vi "Write logEntry.vi"(10 "logEntry":string[](array[string]), 11 "Logger in":refnum<class "Log.lvclass">) -> (3 "Logger out":refnum<class "Log.lvclass">)   [LabVIEW 2013, in "Log.lvlib" / "Log.lvclass"]
uses:
  <userlib>/Common/Log/Log/Log.lvclass
  <userlib>/Common/Log/Log/Log.lvclass/Log.ctl
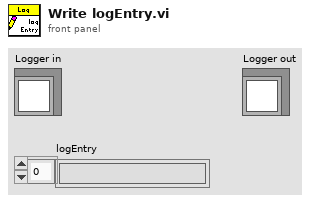
[diagram p1: front panel]
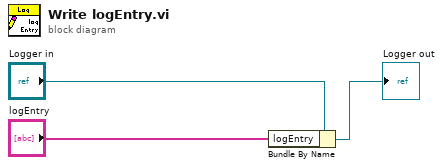
[diagram p0: block diagram]
diagram:
  n1 = Bundle By Name(cluster="Logger in", "logEntry"="logEntry") -> (→"Logger out":refnum<class "Log.lvclass">)
